vi "TurnToAngle.vi"(6 "Invert Direction":bool, 8 "Trigger Range":dbl=12.0, 10 "Turn To":dbl(knob) scale=-180.0..180.0, 11 "Gyro":dbl(knob) scale=-180.0..180.0) -> (0 "Triggered":bool, 2 "Offset Angle":dbl(knob) scale=-180.0..180.0)   [LabVIEW 2018]
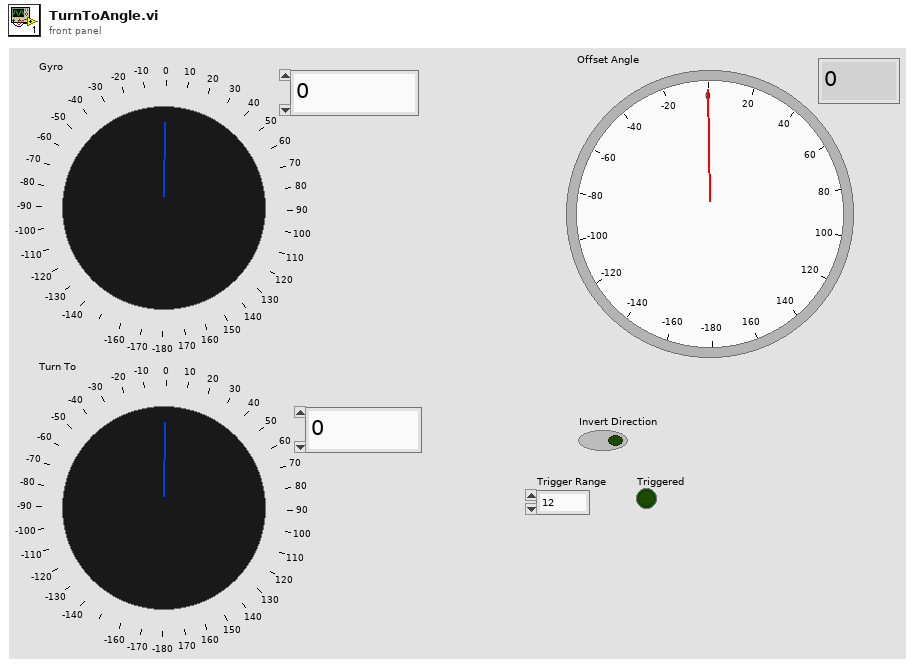
[diagram p1: front panel]
types:
  T1 = enum16{"[0, 360]", "[-180, 180]", "[0, 2PI]", "[-PI, PI]"}
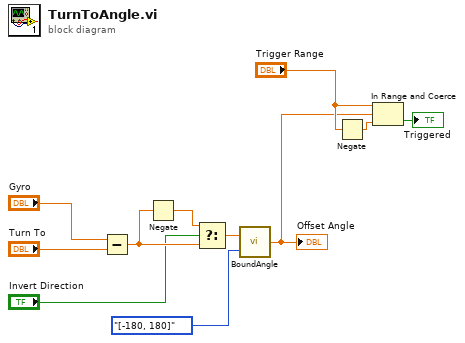
[diagram p0: block diagram]
diagram:
  n1 = Subtract(x="Gyro", y="Turn To") -> (x-y=w7:dbl)
  n2 = Negate(x=w7) -> (-x=w8:dbl)
  n3 = Select(t=w8, s="Invert Direction", f=w7) -> (s? t:f=w5:dbl)
  n4 = call <userlib>:"BoundAngle.vi"("Type"=T1."[-180, 180]", "Angle"=w5) -> ("Bound Angle"=w1:dbl)
  "Offset Angle" <- w1
  n5 = Negate(x="Trigger Range") -> (-x=w4:dbl)
  n6 = In Range and Coerce(upper limit="Trigger Range", x=w1, lower limit=w4) -> (In Range?=→"Triggered":bool)  [unwired: 1 out]
